vi "Set PID Tuning.vi"(8 "error in (no error)":errorcluster, 10 "PID Tuning":T1, 11 "Rover in":refnum<class "Rover.lvclass">) -> (0 "error out":errorcluster, 3 "Rover out":refnum<class "Rover.lvclass">)   [LabVIEW 2020, in "Rover.lvlib" / "Rover.lvclass"]
uses:
  Rover.lvclass
  PID Tuning.ctl
  I2C Register.ctl
  Rover.lvclass/Rover.ctl
  <vilib>/MakerHub/LINX/Private/Local IO/LinxI2cWrite.vi
  <vilib>/MakerHub/LINX/Public/Utilities/Check Channel.vi
  <vilib>/MakerHub/LINX/Private/Local IO/Handle Errors.vi
  <vilib>/MakerHub/LINX/Private/Utilties/Generate Error.vi
  <vilib>/MakerHub/LINX/LMH-LINX.lvlib
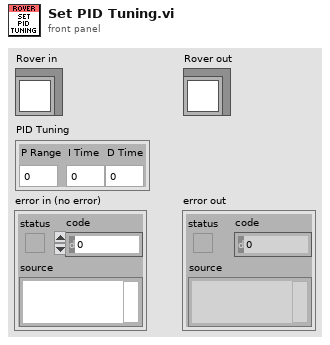
[diagram p1: front panel]
types:
  T1 = typedef "Rover.lvlib/Rover.lvclass/PID Tuning.ctl" = cluster{"P Range":sgl, "I Time":sgl, "D Time":sgl}
  T2 = typedef "Rover.lvlib/Rover.lvclass/I2C Register.ctl" = enum8{"encA", "encB", "ticksPerUnit", "width", "flags", "velP", "velI", "velD", "velMin", "velMax", "poseX", "poseY", "poseA", "cmdDrive", "cmdTurn", "velocity", "turn", "velL", "velR", "run", "outL", "outR", "outDeadband"}
  T3 = typedef "LMH-LINX.lvlib/LINX Ref.ctl" = cluster{"IO":T4, "Interface":T5, "LINX Device Config":T6}
  T4 = typedef "LMH-LINX.lvlib/Platform.ctl" = enum16{"Remote", "Local"}
  T5 = typedef "LMH-LINX.lvlib/Interface.ctl" = enum16{"Serial", "TCP"}
  T6 = typedef "LMH-LINX.lvlib/Device.lvlib/LINX Device Config.ctl" = cluster{"Interface":T5, "COM Port":refnum<visa-resource-name>, "TCP Configuration":T7, "Device Family":u8, "Device ID":u8, "Device Name":string, "TCP Ref":refnum<k5>, "Channels":T8}
  T7 = typedef "LMH-LINX.lvlib/Device.lvlib/TCP Config.ctl" = cluster{"IP Address":string, "Port":u16}
  T8 = typedef "LMH-LINX.lvlib/Channels.ctl" = cluster{"DI":u8[], "DO":u8[], "AI":u8[], "AO":u8[], "PWM":u8[], "QE":u8[], "UART":u8[], "I2C 2":u8[], "SPI":u8[], "CAN":u8[], "Servo":u8[], "AI Ref (V)":dbl, "AI Resolution (Bits)":u8, "AO Ref (V)":dbl, "AO Resolution (Bits)":u8}
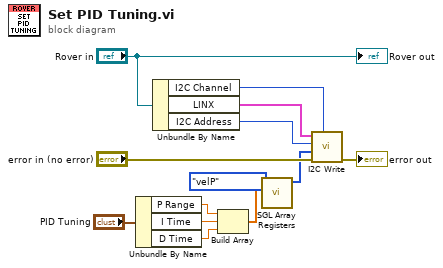
[diagram p0: block diagram]
diagram:
  n1 = Unbundle By Name("PID Tuning") -> ("P Range"=w6:sgl, "I Time"=w5:sgl, "D Time"=w4:sgl)
  n2 = Unbundle By Name("Rover in") -> ("I2C Channel"=w8:u8, "LINX"=w10:T3, "I2C Address"=w9:u8)
  n3 = Build Array(w6, w5, w4) -> (w3:sgl[])
  n4 = call "SGL Array Registers.vi"("SGL Array"=w3, "I2C Register"=I2C_Register."velP") -> ("Data"=w2:u8[])  [unwired: 9 in]
  n5 = call <vilib>:"I2C Write.vi"("I2C Channel"=w8, "Error In"="error in (no error)", "Data"=w2, "I2C Slave Address (0)"=w9, "LINX Resource"=w10) -> ("Error Out"=→"error out":errorcluster)  [unwired: 5 in, 1 out]
  "Rover out" <- "Rover in"
